vi "Get Line Detector Object.vi"() -> (3 "Module":refnum<class "Template Module.lvclass">)   [LabVIEW 2016]
uses:
  Template Module/Template Module.lvclass
  Line Detector.lvclass
  C:/github/LabActor/Template Module/Template Module.lvclass
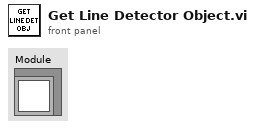
[diagram p1: front panel]
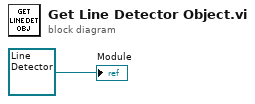
[diagram p0: block diagram]
diagram:
  "Module" <- refnum<class "Line Detector.lvclass"> refnum ("Line Detector.lvclass")
